vi "Run Tool Bar.vi"(9 "Tool Name Text Box":refnum<vi>, 12 "IMAQ Display Refs":refnum<vi>[](array[refnum])) -> ()   [LabVIEW 2016]
panel:
  in  "Exit":bool
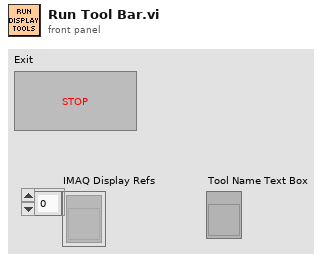
[diagram p1: front panel]
types:
  T1 = enum32{"Invalid", "Standard", "Closed", "Hidden", "Minimized", "Maximized"}
  T2 = enum32{"Bad", "Idle", "Run top level", "Running"}
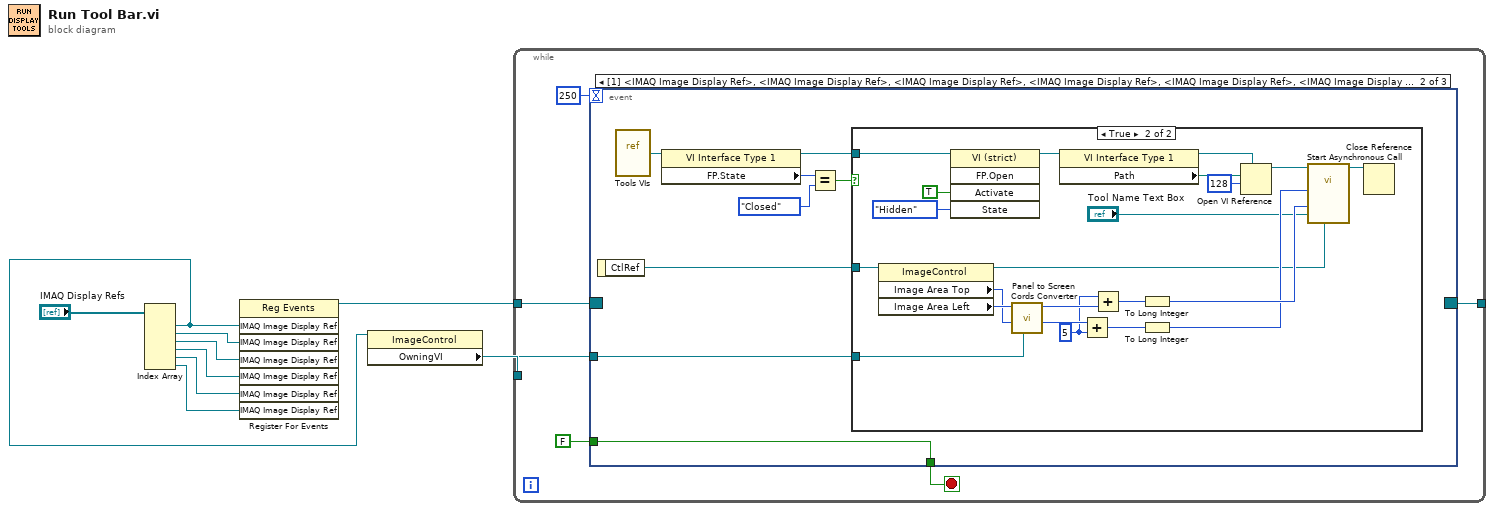
[diagram p0: block diagram]
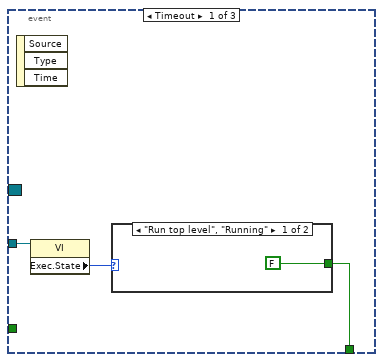
[diagram p2: hidden frame]
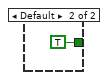
[diagram p3: hidden frame]
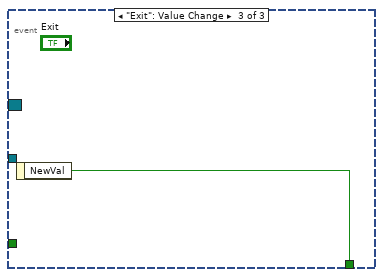
[diagram p5: hidden frame]
diagram:
  n1 = Index Array(array="IMAQ Display Refs") -> (element #1=w3:refnum<vi>, element #2=w8:refnum<vi>, element #3=w5:refnum<vi>, element #4=w6:refnum<vi>, element #5=w7:refnum<vi>, element #6=w4:refnum<vi>)  [unwired: 6 in]
  n2 = register-events(w3, w8, w5, w6, w7, w4) -> (reference out=w2:refnum<event-registration>)  [unwired: 2 in, 1 out]
  n3 = property class="ImageControl"(reference=w3) -> ("OwningVI"=w1:refnum<vi>)  [unwired: 1 in, 2 out]
  n4 = while {
    tunnel: w2 -> [w12]
    tunnel: w1 -> [w11]
    tunnel: [w10] -> _
    stop <- w15 stop-if-true
    n5 = event shown="[1] <IMAQ Image Display Ref>, <IMAQ Image Display Ref>, <IMAQ Image Display Ref>, <IMAQ Image Display Ref>, <IMAQ Image Display Ref>, <IMAQ Image Display Ref>: Mouse Enter" {
      selector: w12 -> [_ _ _]
      dyn-events: [_ _ _] -> w10
      timeout: 250 -> [_ _ _]
      tunnel: [w16 w22 w51] -> w15
      tunnel: FALSE -> [_ w22 _]
      tunnel: w11 -> [w17 w21 _]
      event Timeout {
        n6 = event-data() -> ()  [unwired: 1 in, 3 out]
        n7 = property class="VI"(reference=w17) -> ("Exec.State"=w18:T2)  [unwired: 1 in, 2 out]
        n8 = case shown="\"Run top level\", \"Running\"" w18 {
          tunnel: [FALSE TRUE] -> w16
          frame "Run top level", "Running" {
          }
          frame Default {
          }
        }
      }
      event Mouse Enter {
        n9 = event-data() -> ("CtlRef"=w24:refnum<vi>)  [unwired: 1 in]
        n10 = vi-ref "Tools VIs.vi"() -> (w26:refnum<vi>)
        n11 = property class="VI Interface Type 1"(reference=w26) -> (reference out=w23:refnum<vi>, "FP.State"=w27:T1)  [unwired: 1 in, 1 out]
        n12 = Equal?(x=w27, y=T1."Closed" ("Front Panel Window:State")) -> (x = y?=w25:bool)
        n13 = case shown="True" w25 {
          tunnel: w24 -> [_ w41]
          tunnel: w23 -> [_ w48]
          tunnel: w21 -> [_ w30]
          frame False {
          }
          frame True {
            w34 = i16 5 ("y")
            n14 = property class="ImageControl"(reference=w41) -> (reference out=w31:refnum<vi>, "Image Area Top"=w39:i32, "Image Area Left"=w40:i32)  [unwired: 1 in, 1 out]
            n15 = invoke class="VI (strict)" method="FP.Open"(reference=w48, "Activate"=TRUE ("Activate?"), "State"=T1."Hidden") -> (reference out=w42:refnum<vi>)  [unwired: 2 in, 4 out]
            n16 = call "Panel to Screen Cords Converter.vi"("VI Ref"=w30, "Vertical FP 1"=w39, "Horizontal FP 1"=w40) -> ("Vertical Screen 1"=w38:i16, "Horizontal Screen 1"=w36:i16)  [unwired: 5 in, 2 out]
            n17 = property class="VI Interface Type 1"(reference=w42) -> (reference out=w43:refnum<vi>, "Path"=w47:path)  [unwired: 1 in, 1 out]
            n18 = Add(x=w38, y=w34) -> (x+y=w37:i16)
            n19 = Add(x=w34, y=w36) -> (x+y=w35:i16)
            n20 = To Long Integer(number=w35) -> (32bit integer=w33:i32)
            n21 = To Long Integer(number=w37) -> (32bit integer=w32:i32)
            n22 = Open VI Reference(type specifier VI Refnum (for type only)=w43, vi path=w47, options=128) -> (vi reference=w45:refnum<vi>)  [unwired: 3 in, 1 out]
            n23 = call-by-ref "Start Asynchronous Call"(reference=w45, "IMAQ Image Display Ref"=w31, "Tool Name Text Ref"="Tool Name Text Box", "Left (Screen Coords, px)"=w33, "Top (Screen Coords, px)"=w32) -> (reference out=w44:refnum<vi>)  [unwired: 9 in, 1 out]
            n24 = Close Reference(reference=w44) -> ()  [unwired: 1 in, 1 out]
          }
        }
      }
      event "Exit": Value Change {
        n25 = event-data() -> ("NewVal"=w51:bool)  [unwired: 1 in]
      }
    }
  }
